vi "Lab3_main.vi"() -> ()   [LabVIEW 2020]
panel:
  out "u(t), theta_sim(t), theta_motor(t)":T1(graph)
  out "theta_sim(t), theta_motor(t)":cluster{"Position":dbl, "position (rad)":dbl}(graph)
  in  "System Params":cluster{"b":dbl, "a0":dbl, "a1":dbl, "a2":dbl}
  in  "Frequency":dbl
  in  "Amplitude":dbl
  in  "Signal Type":u16(ring) items=["square", "triangle", "sinusoidal"]
  out "u(t), u_motor(t), theta_motor(t)":T2(graph)
  in  "dt [s]":dbl
  in  "On/Off":bool
  out "?":bool
  in  "stop":bool
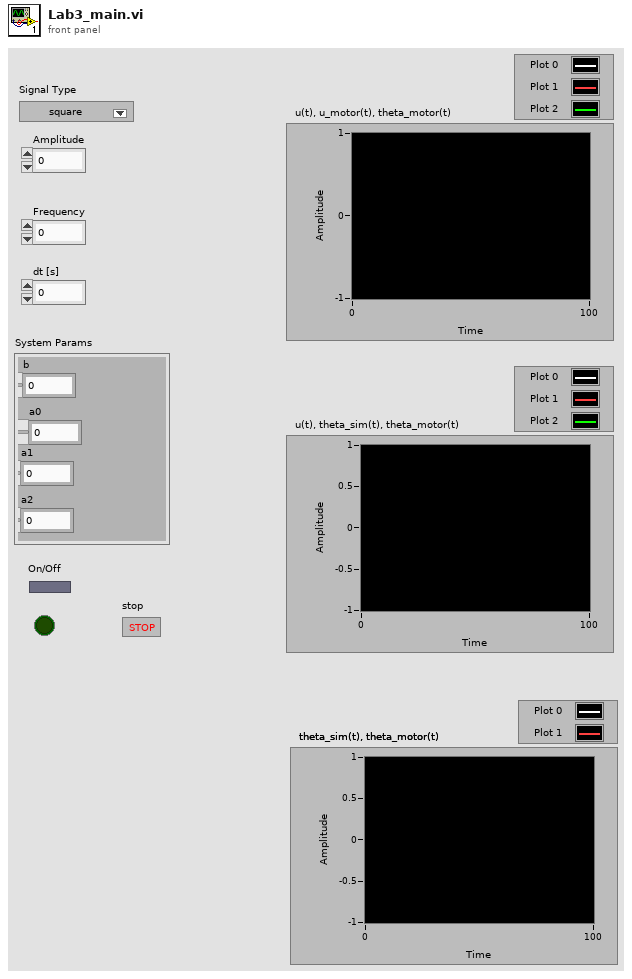
[diagram p1: front panel]
types:
  T1 = cluster{"Signal":dbl, "Position":dbl, "position (rad)":dbl}
  T2 = cluster{"Signal":dbl, "Vm (V)":dbl, "position (rad)":dbl}
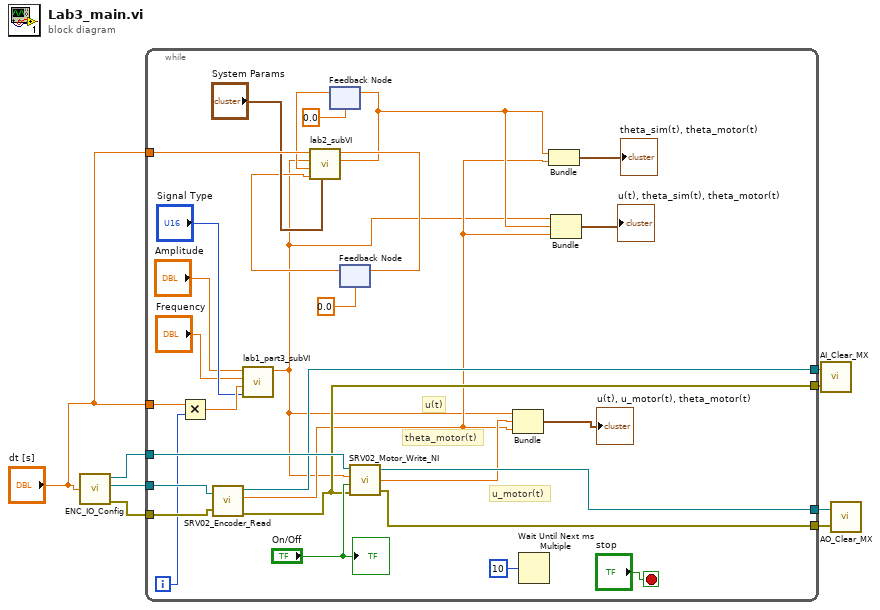
[diagram p0: block diagram]
diagram:
  n1 = call "ENC_IO_Config.vi"("dt"="dt [s]") -> ("AO Task"=w8:refnum<k21>, "ENC Task"=w7:refnum<k21>, "IO error out"=w6:errorcluster)  [unwired: 2 in, 1 out]
  n2 = while {
    tunnel: w8 -> [w33]
    tunnel: w7 -> [w35]
    tunnel: w6 -> [w36]
    tunnel: [w32] -> w5
    tunnel: [w31] -> w4
    tunnel: [w30] -> w3
    tunnel: [w29] -> w2
    tunnel: "dt [s]" -> [w26]
    tunnel: "dt [s]" -> [w20]
    i -> [w27]
    stop <- "stop" stop-if-true
    # "u(t)"
    # "theta_motor(t)"
    # "u_motor(t)"
    n3 = Multiply(x=w26, y=w27) -> (x*y=w28:dbl)
    n4 = call "SRV02_Encoder_Read.vi"("task/channels in"=w35, "error in"=w36) -> ("task out"=w29:refnum<k21>, "position (rad)"=w10:dbl, "error out"=w30:errorcluster)  [unwired: 1 out]
    n5 = call "lab1_part3_subVI.vi"("Signal Type"="Signal Type", "Time"=w28, "Frequency"="Frequency", "Amplitude"="Amplitude") -> ("Signal"=w9:dbl)  [unwired: 7 in]
    n6 = feedback #1(0.0) -> (w18:dbl)
    n7 = feedback #2(0.0) -> (w16:dbl)
    n8 = call "lab2_subVI.vi"("System Params"="System Params", "Velocity"=w16, "Position"=w18, "Input"=w9, "dt"=w20) -> ("Position"=w11:dbl, "Velocity"=w17:dbl)  [unwired: 5 in]
    n9 = feedback-in #1(w11) -> ()
    n10 = feedback-in #2(w17) -> ()
    n11 = call "SRV02_Motor_Write_NI.vi"("error in"=w30, "operate?"="On/Off", "u (V)"=w9, "task in"=w33) -> ("error out"=w32:errorcluster, "Vm (V)"=w24:dbl, "task out"=w31:refnum<k21>)
    n12 = Bundle("Signal"=w9, "Vm (V)"=w24, "position (rad)"=w10) -> (→"u(t), u_motor(t), theta_motor(t)":T2)  [unwired: 1 in]
    n13 = Wait Until Next ms Multiple(millisecond multiple=10) -> ()  [unwired: 1 out]
    n14 = Bundle("Position"=w11, "position (rad)"=w10) -> (→"theta_sim(t), theta_motor(t)":cluster{"Position":dbl, "position (rad)":dbl})  [unwired: 1 in]
    n15 = Bundle("Signal"=w9, "Position"=w11, "position (rad)"=w10) -> (→"u(t), theta_sim(t), theta_motor(t)":T1)  [unwired: 1 in]
    "?" <- "On/Off"
  }
  n16 = call "AI_Clear_MX.vi"("Error in"=w3, "Task in"=w2) -> ()  [unwired: 1 out]
  n17 = call "AO_Clear_MX.vi"("Error in"=w5, "Task in"=w4) -> ()  [unwired: 1 out]
